vi "Main.vi"() -> ()   [LabVIEW 2021]
doc: "The myRIO Project template acquires acceleration data from the onboard accelerometer and displays the changes of acceleration values in a waveform chart."
uses:
  <vilib>/userDefined/High Color/IMAQdx.ctl
  <vilib>/myRIO/Common/Instrument Driver Framework/myRIO v1.0/UART/vis/myRIO v1.0 Close UART.vi
  <vilib>/myRIO/Common/Instrument Driver Framework/Utilities/vis/FPGA Ref Manager.vi
  <vilib>/myRIO/Common/Instrument Driver Framework/myRIO v1.0/myRIO v1.0 Reset FPGA.vi
  <vilib>/myRIO/Common/Instrument Driver Framework/myRIO v1.0/IRQ/vis/myRIO v1.0 IRQ Info FGV.vi
  <vilib>/myRIO/Common/Instrument Driver Framework/myRIO v1.0/IRQ/vis/myRIO v1.0 Timer IRQ Info FGV.vi
  <vilib>/myRIO/Common/Instrument Driver Framework/myRIO v1.0/IRQ/vis/myRIO v1.0 ISR Agent.vi
  <vilib>/myRIO/Instrument Drivers/Utilities/vis/Reset Index.vi
  <vilib>/myRIO/Common/Instrument Driver Framework/myRIO v1.0/Resource Manager/vis/myRIO v1.0 Block Write Resource Manager.vi
  <vilib>/myRIO/Instrument Drivers/Utilities/Utilities.lvlib
panel:
  in  "Stepper Two":i32=-5
  in  "Stepper One":i32=-5
  out "Position":cluster{"X":sgl, "Y":sgl}
  out "error out":errorcluster
  # "Overview: The myRIO Project template acquires acceleration data from the onboard accelerometer and displays the changes of acceleration values in a waveform chart.\nInstructions:\n1. Check the myRIO target IP address in the project and make sure the target IP address is correct. \n2. Run this VI."
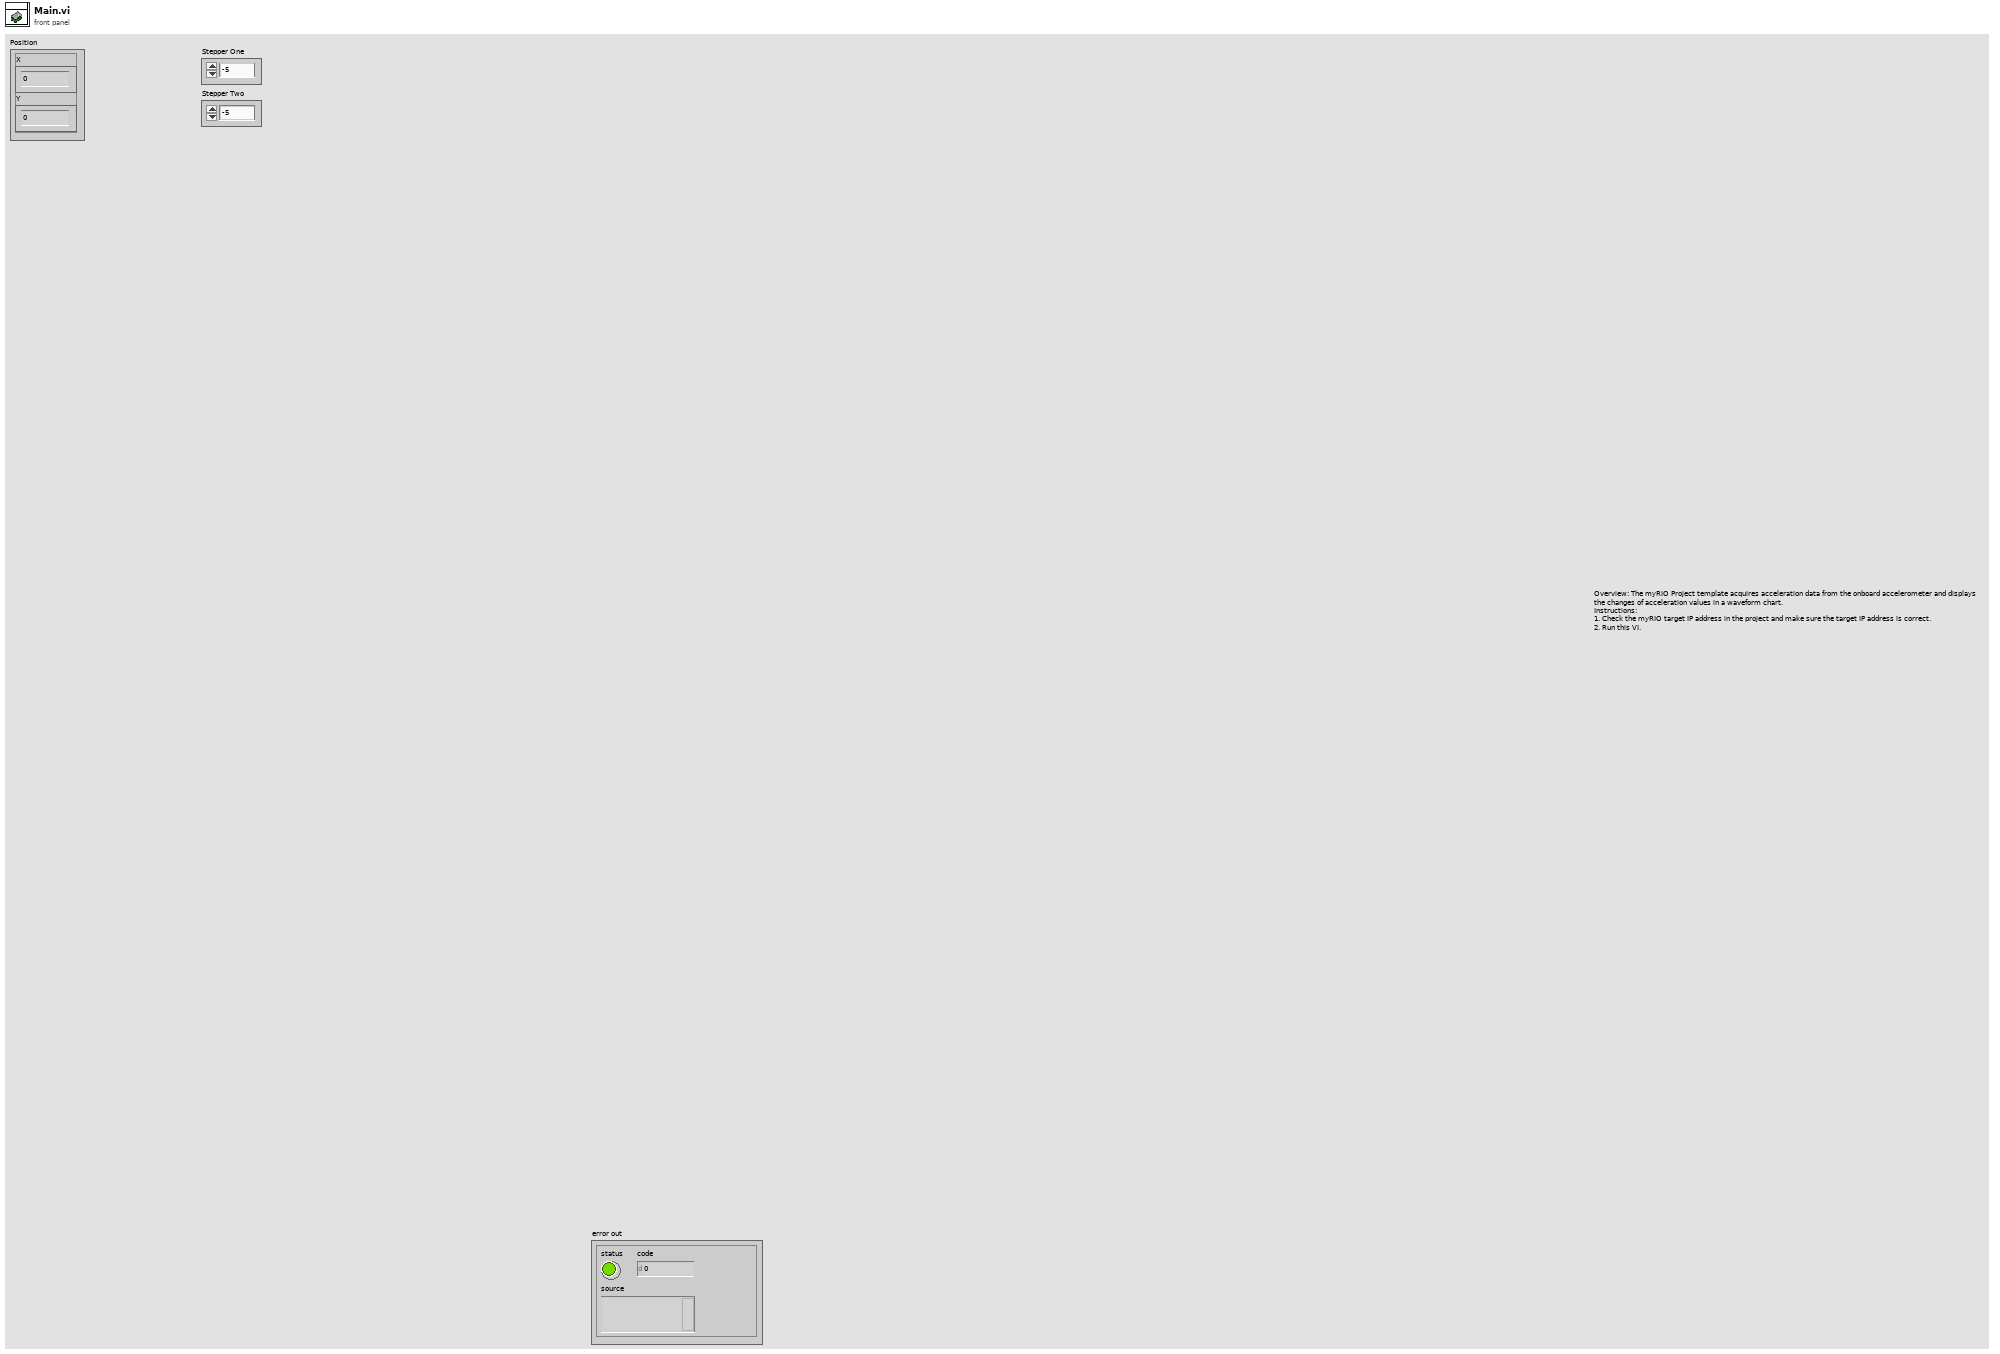
[diagram p1: front panel]
types:
  T1 = typedef "IMAQdx.ctl" = refnum<k21>
  T2 = typedef "IMAQ Image.ctl" = refnum<image>
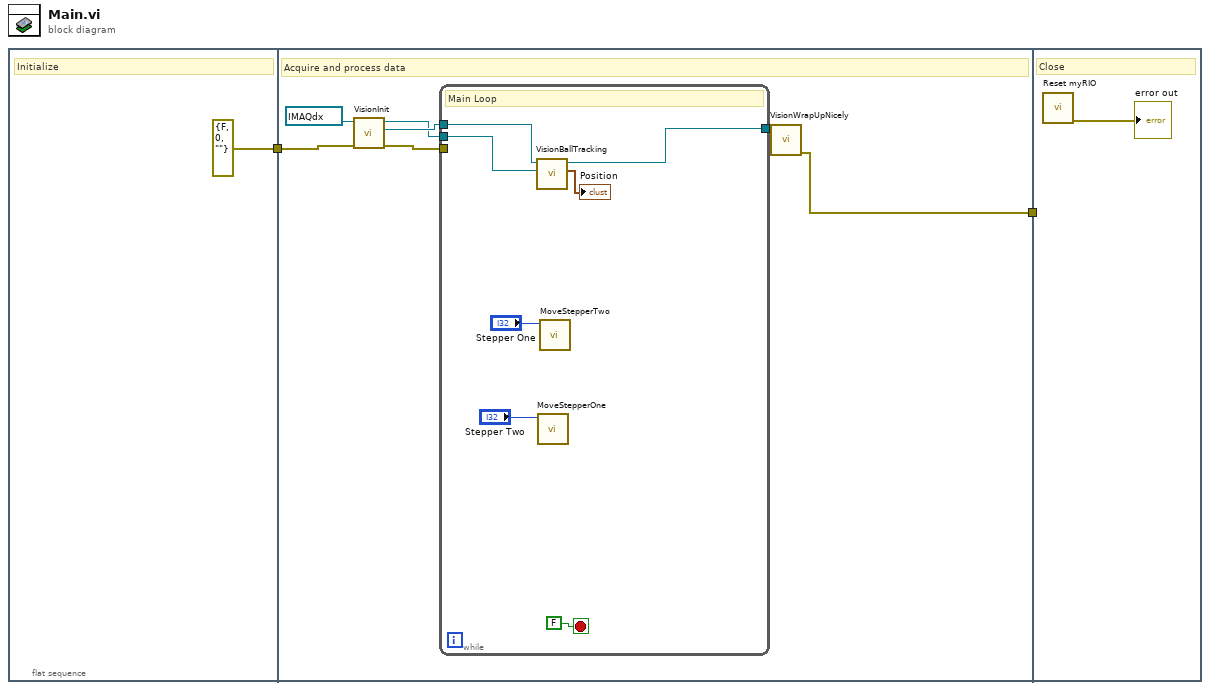
[diagram p0: block diagram]
diagram:
  n1 = flat-sequence {
    tunnel: [errorcluster {"status"=FALSE, "code"=0, "source"=""} ("error in")] -> w2
    tunnel: w2 -> [w6]
    tunnel: [w5] -> w1
    tunnel: w1 -> [_]
    frame #0 {
      # "Initialize"
    }
    frame #1 {
      # "Acquire and process data"
      n2 = call "VisionInit.vi"("error in (no error)"=w6, "Refnum in"=T1 "cam0") -> ("error out"=w7:errorcluster, "New Image"=w10:T2, "Refnum out"=w8:T1)  [unwired: 7 in]
      n3 = while {
        tunnel: w8 -> [w15]
        tunnel: w7 -> [_]
        tunnel: [w17] -> w9
        tunnel: w10 -> [w14]
        stop <- FALSE stop-if-true
        # "Main Loop"
        n4 = call "VisionBallTracking.vi"(10:"Refnum in"=w15, 11:"Refnum in"=w14) -> ("Position"=→"Position":cluster{"X":sgl, "Y":sgl}, "Refnum out"=w17:T1)  [unwired: 8 in]
        n5 = call "MoveStepperOne.vi"("Numeric"="Stepper Two") -> ()  [unwired: 11 in]
        n6 = call "MoveStepperTwo.vi"("Numeric"="Stepper One") -> ()  [unwired: 11 in]
      }
      n7 = call "VisionWrapUpNicely.vi"("Refnum in"=w9) -> ("error out"=w5:errorcluster)  [unwired: 10 in]
    }
    frame #2 {
      # "Close"
      n8 = call <vilib>:"Reset myRIO.vi"() -> ("error out"=→"error out":errorcluster)  [unwired: 11 in]
    }
  }
